vi "M14 Turret_Hardware_Globals.vi"() -> ()   [LabVIEW 2019]
panel:
  in  "Turret_Spark_Motor_A":string="Turret_Spark_Motor_A"
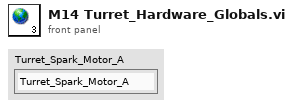
[diagram p1: front panel]
diagram:
